vi "guangzi - 可控采集.vi"() -> ()   [LabVIEW 2016]
uses:
  <vilib>/Utility/file.llb/Write To Spreadsheet File (DBL).vi
panel:
  in  "采集记录开关":bool
  out "切片图":u32[](graph)
  in  "切片值":i32
  in  "选项卡控件":T1(tab)
  in  "对数":bool
  out "MCS8Dat Error":i32
  out "CHN Status":T2 {"Dummy" format="%.2f"; "Starts" format="%.2f"; "Sweeps" format="%.2f"; "Roirate" format="%.2f"; "RoiSum" format="%.2f"; "TotalSum" format="%.2f"; "Fifo full" format="%.2f"; "Runtime" format="%.2f"}
  out "Data":u32[](graph)
  out "Settings":T3 {"dummy3" format="%.2f"; "dummy2" format="%.2f"; "bitshift" format="%.0x"; "Active" format="%.0x"; "Offset" format="%.0x"; "Param" format="%.0x"; "dummy1" format="%.2f"; "Roipreset" format="%.2f"; "cftfak" format="%.0x"}
  out "通道数":i32
  out "Data 9":dbl[](graph)
  out "Data 2":u32[](graph)
  out "MCS8Dat Error 2":i32
  out "Settings 2":T3 {"dummy3" format="%.2f"; "dummy2" format="%.2f"; "bitshift" format="%.0x"; "Active" format="%.0x"; "Offset" format="%.0x"; "Param" format="%.0x"; "dummy1" format="%.2f"; "Roipreset" format="%.2f"; "cftfak" format="%.0x"}
  out "CHN Status 2":T2 {"Dummy" format="%.2f"; "Starts" format="%.2f"; "Sweeps" format="%.2f"; "Roirate" format="%.2f"; "RoiSum" format="%.2f"; "TotalSum" format="%.2f"; "Fifo full" format="%.2f"; "Runtime" format="%.2f"}
  out "通道数 2":i32
  in  "对数 2":bool
  out "Data10":dbl[](graph)
  out "Data 3":u32[](graph)
  out "MCS8Dat Error 3":i32
  out "Settings 3":T3 {"dummy3" format="%.2f"; "dummy2" format="%.2f"; "bitshift" format="%.0x"; "Active" format="%.0x"; "Offset" format="%.0x"; "Param" format="%.0x"; "dummy1" format="%.2f"; "Roipreset" format="%.2f"; "cftfak" format="%.0x"}
  out "CHN Status 3":T2 {"Dummy" format="%.2f"; "Starts" format="%.2f"; "Sweeps" format="%.2f"; "Roirate" format="%.2f"; "RoiSum" format="%.2f"; "TotalSum" format="%.2f"; "Fifo full" format="%.2f"; "Runtime" format="%.2f"}
  out "通道数 3":i32
  in  "对数 3":bool
  out "Data10 2":dbl[](graph)
  out "Data 4":u32[](graph)
  out "MCS8Dat Error 4":i32
  out "Settings 4":T3 {"dummy3" format="%.2f"; "dummy2" format="%.2f"; "bitshift" format="%.0x"; "Active" format="%.0x"; "Offset" format="%.0x"; "Param" format="%.0x"; "dummy1" format="%.2f"; "Roipreset" format="%.2f"; "cftfak" format="%.0x"}
  out "CHN Status 4":T2 {"Dummy" format="%.2f"; "Starts" format="%.2f"; "Sweeps" format="%.2f"; "Roirate" format="%.2f"; "RoiSum" format="%.2f"; "TotalSum" format="%.2f"; "Fifo full" format="%.2f"; "Runtime" format="%.2f"}
  out "通道数 4":i32
  in  "对数 4":bool
  out "Data10 3":dbl[](graph)
  out "Data 5":u32[](graph)
  out "MCS8Dat Error 5":i32
  out "Settings 5":T3 {"dummy3" format="%.2f"; "dummy2" format="%.2f"; "bitshift" format="%.0x"; "Active" format="%.0x"; "Offset" format="%.0x"; "Param" format="%.0x"; "dummy1" format="%.2f"; "Roipreset" format="%.2f"; "cftfak" format="%.0x"}
  out "CHN Status 5":T2 {"Dummy" format="%.2f"; "Starts" format="%.2f"; "Sweeps" format="%.2f"; "Roirate" format="%.2f"; "RoiSum" format="%.2f"; "TotalSum" format="%.2f"; "Fifo full" format="%.2f"; "Runtime" format="%.2f"}
  out "通道数 5":i32
  in  "对数 5":bool
  out "Data10 4":dbl[](graph)
  out "Data 6":u32[](graph)
  out "MCS8Dat Error 6":i32
  out "Settings 6":T3 {"dummy3" format="%.2f"; "dummy2" format="%.2f"; "bitshift" format="%.0x"; "Active" format="%.0x"; "Offset" format="%.0x"; "Param" format="%.0x"; "dummy1" format="%.2f"; "Roipreset" format="%.2f"; "cftfak" format="%.0x"}
  out "CHN Status 6":T2 {"Dummy" format="%.2f"; "Starts" format="%.2f"; "Sweeps" format="%.2f"; "Roirate" format="%.2f"; "RoiSum" format="%.2f"; "TotalSum" format="%.2f"; "Fifo full" format="%.2f"; "Runtime" format="%.2f"}
  out "通道数 6":i32
  in  "对数 6":bool
  out "Data10 5":dbl[](graph)
  out "Data 7":u32[](graph)
  out "MCS8Dat Error 7":i32
  out "Settings 7":T3 {"dummy3" format="%.2f"; "dummy2" format="%.2f"; "bitshift" format="%.0x"; "Active" format="%.0x"; "Offset" format="%.0x"; "Param" format="%.0x"; "dummy1" format="%.2f"; "Roipreset" format="%.2f"; "cftfak" format="%.0x"}
  out "CHN Status 7":T2 {"Dummy" format="%.2f"; "Starts" format="%.2f"; "Sweeps" format="%.2f"; "Roirate" format="%.2f"; "RoiSum" format="%.2f"; "TotalSum" format="%.2f"; "Fifo full" format="%.2f"; "Runtime" format="%.2f"}
  out "通道数 7":i32
  in  "对数 7":bool
  out "Data10 6":dbl[](graph)
  out "Data 8":u32[](graph)
  out "MCS8Dat Error 8":i32
  out "Settings 8":T3 {"dummy3" format="%.2f"; "dummy2" format="%.2f"; "bitshift" format="%.0x"; "Active" format="%.0x"; "Offset" format="%.0x"; "Param" format="%.0x"; "dummy1" format="%.2f"; "Roipreset" format="%.2f"; "cftfak" format="%.0x"}
  out "CHN Status 8":T2 {"Dummy" format="%.2f"; "Starts" format="%.2f"; "Sweeps" format="%.2f"; "Roirate" format="%.2f"; "RoiSum" format="%.2f"; "TotalSum" format="%.2f"; "Fifo full" format="%.2f"; "Runtime" format="%.2f"}
  out "通道数 8":i32
  in  "对数 8":bool
  out "Data10 7":dbl[](graph)
  in  "子开关":bool
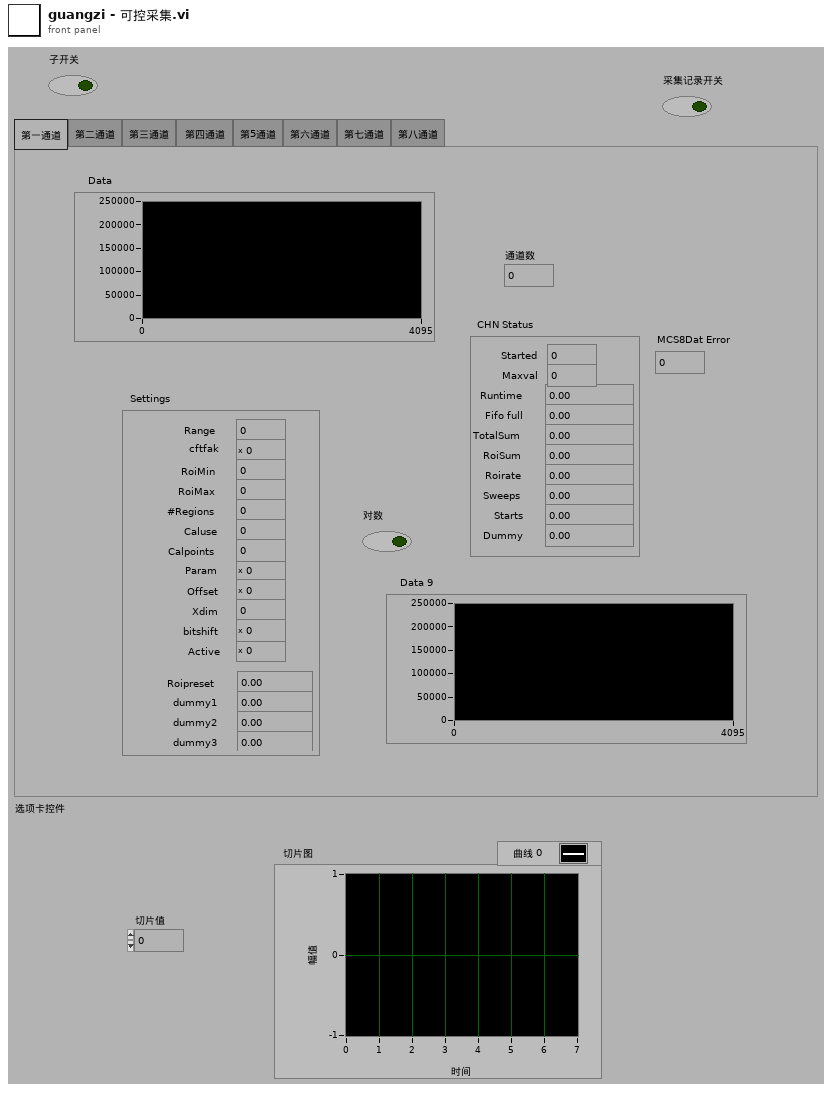
[diagram p1: front panel]
types:
  T1 = enum32{"第一通道", "第二通道", "第三通道", "第四通道 ", "第5通道", "第六通道", "第七通道", "第八通道"}
  T2 = cluster{"Started":i32, "Maxval":u32, "Runtime":dbl, "Fifo full":dbl, "TotalSum":dbl, "RoiSum":dbl, "Roirate":dbl, "Sweeps":dbl, "Starts":dbl, "Dummy":dbl}
  T3 = cluster{"Range":i32, "cftfak":i32, "RoiMin":i32, "RoiMax":i32, "#Regions":i32, "Caluse":i32, "Calpoints":i32, "Param":i32, "Offset":i32, "Xdim":i32, "bitshift":i32, "Active":i32, "Roipreset":dbl, "dummy1":dbl, "dummy2":dbl, "dummy3":dbl}
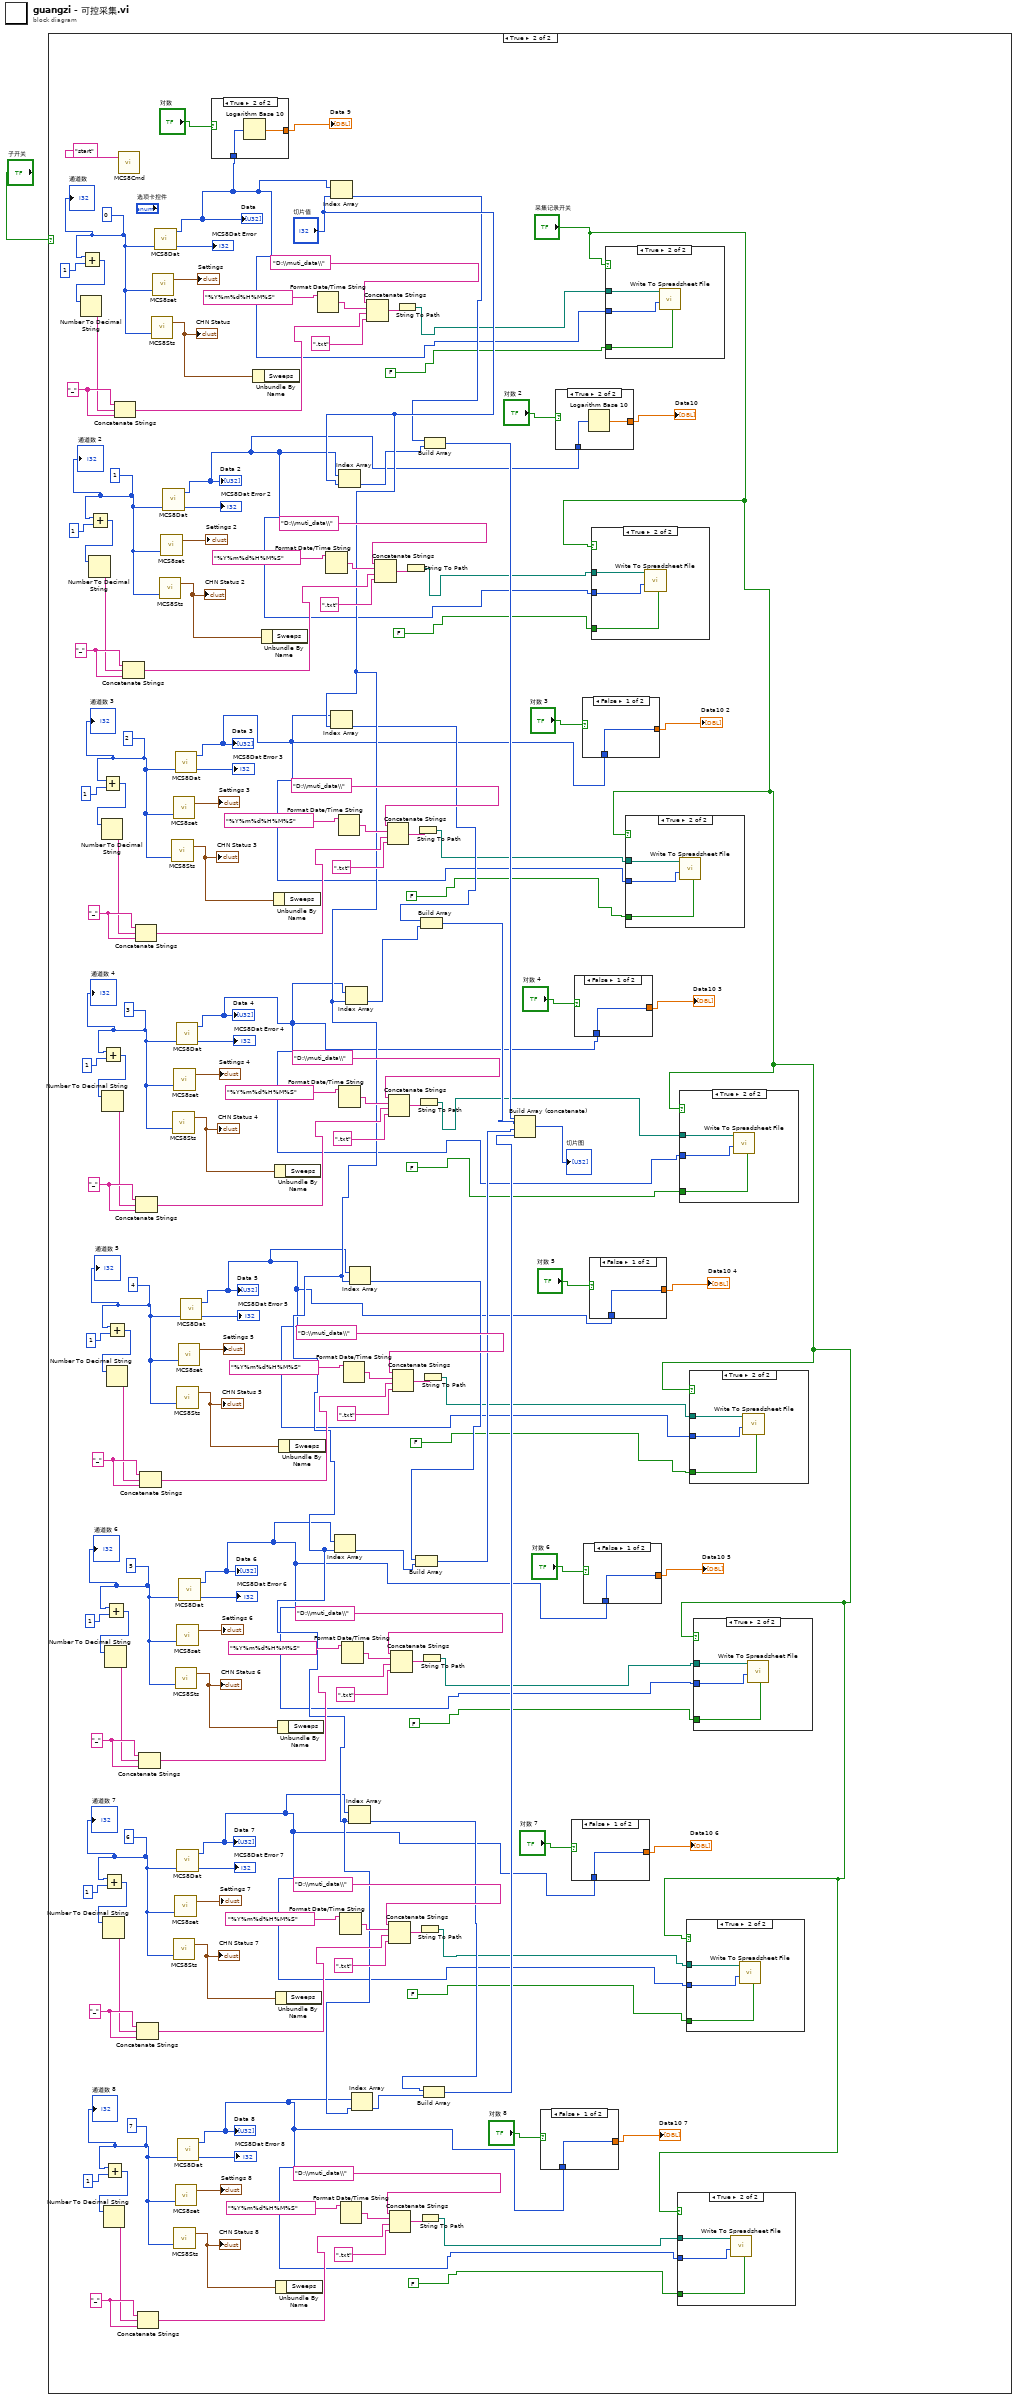
[diagram p0: block diagram]
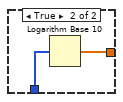
[diagram p11: hidden frame]
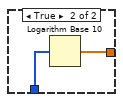
[diagram p12: hidden frame]
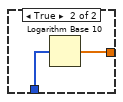
[diagram p13: hidden frame]
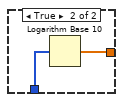
[diagram p14: hidden frame]
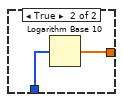
[diagram p15: hidden frame]
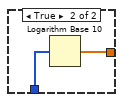
[diagram p16: hidden frame]
diagram:
  n1 = case shown="True" "子开关" {
    frame False {
    }
    frame True {
      w57 = 7
      w65 = "_"
      w71 = 6
      w79 = "_"
      w85 = 5
      w93 = "_"
      w99 = 4
      w107 = "_"
      w113 = 3
      w121 = "_"
      w127 = 2
      w135 = "_"
      w141 = 1
      w149 = "_"
      w155 = 0
      w163 = "_"
      n2 = Add(x=w155, y=1) -> (x+y=w158:i32)
      n3 = Number To Decimal String(number=w158) -> (decimal integer string=w162:string)  [unwired: 1 in]
      n4 = Add(x=w141, y=1) -> (x+y=w144:i32)
      n5 = Number To Decimal String(number=w144) -> (decimal integer string=w148:string)  [unwired: 1 in]
      n6 = Add(x=w127, y=1) -> (x+y=w130:i32)
      n7 = Number To Decimal String(number=w130) -> (decimal integer string=w134:string)  [unwired: 1 in]
      n8 = Add(x=w113, y=1) -> (x+y=w116:i32)
      n9 = Number To Decimal String(number=w116) -> (decimal integer string=w120:string)  [unwired: 1 in]
      n10 = Add(x=w71, y=1) -> (x+y=w74:i32)
      n11 = Number To Decimal String(number=w74) -> (decimal integer string=w78:string)  [unwired: 1 in]
      n12 = Add(x=w57, y=1) -> (x+y=w60:i32)
      n13 = Number To Decimal String(number=w60) -> (decimal integer string=w64:string)  [unwired: 1 in]
      n14 = Add(x=w85, y=1) -> (x+y=w88:i32)
      n15 = Number To Decimal String(number=w88) -> (decimal integer string=w92:string)  [unwired: 1 in]
      n16 = Add(x=w99, y=1) -> (x+y=w102:i32)
      n17 = Number To Decimal String(number=w102) -> (decimal integer string=w106:string)  [unwired: 1 in]
      n18 = Concatenate Strings(w163, w162, w163) -> (w161:string)
      n19 = call "MCS8Cmd.vi"("Command"="start") -> ()  [unwired: 2 in, 1 out]
      n20 = Concatenate Strings(w149, w148, w149) -> (w147:string)
      n21 = Concatenate Strings(w135, w134, w135) -> (w133:string)
      n22 = Concatenate Strings(w121, w120, w121) -> (w119:string)
      n23 = Concatenate Strings(w79, w78, w79) -> (w77:string)
      n24 = Concatenate Strings(w65, w64, w65) -> (w63:string)
      n25 = Concatenate Strings(w93, w92, w93) -> (w91:string)
      n26 = Concatenate Strings(w107, w106, w107) -> (w105:string)
      n27 = call "MCS8Sts.vi"("CHN #"=w155) -> ("CHN Status"=w168:T2)  [unwired: 1 in, 1 out]
      "CHN Status" <- w168
      n28 = call "MCS8set.vi"("Spect #"=w155) -> ("Settings"=→"Settings":T3)  [unwired: 1 in, 1 out]
      n29 = call "MCS8Dat.vi"("Spectrum #"=w155) -> ("MCS8Dat Error"=→"MCS8Dat Error":i32, "Data"=w25:u32[])  [unwired: 2 in, 1 out]
      "Data" <- w25
      n30 = call "MCS8Sts.vi"("CHN #"=w141) -> ("CHN Status"=w154:T2)  [unwired: 1 in, 1 out]
      "CHN Status 2" <- w154
      n31 = call "MCS8set.vi"("Spect #"=w141) -> ("Settings"=→"Settings 2":T3)  [unwired: 1 in, 1 out]
      n32 = call "MCS8Dat.vi"("Spectrum #"=w141) -> ("MCS8Dat Error"=→"MCS8Dat Error 2":i32, "Data"=w22:u32[])  [unwired: 2 in, 1 out]
      "Data 2" <- w22
      n33 = call "MCS8Sts.vi"("CHN #"=w127) -> ("CHN Status"=w140:T2)  [unwired: 1 in, 1 out]
      "CHN Status 3" <- w140
      n34 = call "MCS8Sts.vi"("CHN #"=w113) -> ("CHN Status"=w126:T2)  [unwired: 1 in, 1 out]
      "CHN Status 4" <- w126
      n35 = call "MCS8set.vi"("Spect #"=w127) -> ("Settings"=→"Settings 3":T3)  [unwired: 1 in, 1 out]
      n36 = call "MCS8Sts.vi"("CHN #"=w71) -> ("CHN Status"=w84:T2)  [unwired: 1 in, 1 out]
      "CHN Status 7" <- w84
      n37 = call "MCS8set.vi"("Spect #"=w113) -> ("Settings"=→"Settings 4":T3)  [unwired: 1 in, 1 out]
      n38 = call "MCS8Sts.vi"("CHN #"=w57) -> ("CHN Status"=w70:T2)  [unwired: 1 in, 1 out]
      "CHN Status 8" <- w70
      n39 = call "MCS8set.vi"("Spect #"=w71) -> ("Settings"=→"Settings 7":T3)  [unwired: 1 in, 1 out]
      n40 = call "MCS8Dat.vi"("Spectrum #"=w127) -> ("MCS8Dat Error"=→"MCS8Dat Error 3":i32, "Data"=w19:u32[])  [unwired: 2 in, 1 out]
      "Data 3" <- w19
      n41 = call "MCS8Sts.vi"("CHN #"=w85) -> ("CHN Status"=w98:T2)  [unwired: 1 in, 1 out]
      "CHN Status 6" <- w98
      n42 = call "MCS8set.vi"("Spect #"=w57) -> ("Settings"=→"Settings 8":T3)  [unwired: 1 in, 1 out]
      n43 = call "MCS8Dat.vi"("Spectrum #"=w113) -> ("MCS8Dat Error"=→"MCS8Dat Error 4":i32, "Data"=w15:u32[])  [unwired: 2 in, 1 out]
      "Data 4" <- w15
      n44 = call "MCS8Sts.vi"("CHN #"=w99) -> ("CHN Status"=w112:T2)  [unwired: 1 in, 1 out]
      "CHN Status 5" <- w112
      n45 = call "MCS8set.vi"("Spect #"=w85) -> ("Settings"=→"Settings 6":T3)  [unwired: 1 in, 1 out]
      n46 = call "MCS8Dat.vi"("Spectrum #"=w71) -> ("MCS8Dat Error"=→"MCS8Dat Error 7":i32, "Data"=w7:u32[])  [unwired: 2 in, 1 out]
      "Data 7" <- w7
      n47 = call "MCS8Dat.vi"("Spectrum #"=w57) -> ("MCS8Dat Error"=→"MCS8Dat Error 8":i32, "Data"=w3:u32[])  [unwired: 2 in, 1 out]
      "Data 8" <- w3
      n48 = call "MCS8set.vi"("Spect #"=w99) -> ("Settings"=→"Settings 5":T3)  [unwired: 1 in, 1 out]
      n49 = call "MCS8Dat.vi"("Spectrum #"=w85) -> ("MCS8Dat Error"=→"MCS8Dat Error 6":i32, "Data"=w10:u32[])  [unwired: 2 in, 1 out]
      "Data 6" <- w10
      n50 = call "MCS8Dat.vi"("Spectrum #"=w99) -> ("MCS8Dat Error"=→"MCS8Dat Error 5":i32, "Data"=w13:u32[])  [unwired: 2 in, 1 out]
      "Data 5" <- w13
      n51 = case shown="True" "对数" {
        tunnel: w25 -> [w215 w217]
        tunnel: [w215 w216] -> w41
        frame False {
        }
        frame True {
          n52 = Logarithm Base 10(1:w217) -> (0:w216:dbl[])
        }
      }
      "Data 9" <- w41
      n53 = Unbundle By Name(w168) -> ()  [unwired: 1 out]
      n54 = Unbundle By Name(w154) -> ()  [unwired: 1 out]
      n55 = Unbundle By Name(w140) -> ()  [unwired: 1 out]
      n56 = Unbundle By Name(w126) -> ()  [unwired: 1 out]
      n57 = Unbundle By Name(w84) -> ()  [unwired: 1 out]
      n58 = Unbundle By Name(w70) -> ()  [unwired: 1 out]
      n59 = Unbundle By Name(w98) -> ()  [unwired: 1 out]
      n60 = Unbundle By Name(w112) -> ()  [unwired: 1 out]
      n61 = Format Date/Time String(time format string (%c)="%Y%m%d%H%M%S") -> (date/time string=w159:string)  [unwired: 2 in]
      n62 = Format Date/Time String(time format string (%c)="%Y%m%d%H%M%S") -> (date/time string=w145:string)  [unwired: 2 in]
      n63 = Index Array(array=w25, index="切片值") -> (element=w49:u32)
      n64 = Index Array(array=w19, index="切片值") -> (element=w51:u32)
      n65 = Index Array(array=w10, index="切片值") -> (element=w53:u32)
      n66 = Format Date/Time String(time format string (%c)="%Y%m%d%H%M%S") -> (date/time string=w131:string)  [unwired: 2 in]
      n67 = Index Array(array=w22, index="切片值") -> (element=w48:u32)
      n68 = Format Date/Time String(time format string (%c)="%Y%m%d%H%M%S") -> (date/time string=w117:string)  [unwired: 2 in]
      n69 = Format Date/Time String(time format string (%c)="%Y%m%d%H%M%S") -> (date/time string=w75:string)  [unwired: 2 in]
      n70 = Format Date/Time String(time format string (%c)="%Y%m%d%H%M%S") -> (date/time string=w61:string)  [unwired: 2 in]
      n71 = Format Date/Time String(time format string (%c)="%Y%m%d%H%M%S") -> (date/time string=w89:string)  [unwired: 2 in]
      n72 = Format Date/Time String(time format string (%c)="%Y%m%d%H%M%S") -> (date/time string=w103:string)  [unwired: 2 in]
      n73 = Index Array(array=w15, index="切片值") -> (element=w50:u32)
      n74 = Index Array(array=w7, index="切片值") -> (element=w54:u32)
      n75 = Index Array(array=w13, index="切片值") -> (element=w52:u32)
      n76 = Index Array(array=w3, index="切片值") -> (element=w55:u32)
      n77 = Concatenate Strings("D:\\muti_data\\", w159, w161, ".txt") -> (w165:string)
      n78 = Concatenate Strings("D:\\muti_data\\", w145, w147, ".txt") -> (w151:string)
      n79 = Concatenate Strings("D:\\muti_data\\", w131, w133, ".txt") -> (w137:string)
      n80 = Concatenate Strings("D:\\muti_data\\", w117, w119, ".txt") -> (w123:string)
      n81 = Concatenate Strings("D:\\muti_data\\", w75, w77, ".txt") -> (w81:string)
      n82 = Concatenate Strings("D:\\muti_data\\", w61, w63, ".txt") -> (w67:string)
      n83 = Concatenate Strings("D:\\muti_data\\", w89, w91, ".txt") -> (w95:string)
      n84 = Concatenate Strings("D:\\muti_data\\", w103, w105, ".txt") -> (w109:string)
      n85 = String To Path(string=w165) -> (path=w26:path)
      n86 = String To Path(string=w151) -> (path=w23:path)
      n87 = Build Array(w52, w53) -> (w45:u32[])
      n88 = String To Path(string=w137) -> (path=w20:path)
      n89 = String To Path(string=w123) -> (path=w17:path)
      n90 = String To Path(string=w81) -> (path=w8:path)
      n91 = String To Path(string=w67) -> (path=w4:path)
      n92 = Build Array(w51, w50) -> (w46:u32[])
      n93 = String To Path(string=w95) -> (path=w11:path)
      n94 = String To Path(string=w109) -> (path=w14:path)
      n95 = Build Array(w54, w55) -> (w44:u32[])
      n96 = Build Array(w49, w48) -> (w47:u32[])
      n97 = Build Array (concatenate)(w47, w46, w45, w44) -> (→"切片图":u32[])
      n98 = case shown="False" "对数 8" {
        tunnel: w3 -> [w194 w196]
        tunnel: [w194 w195] -> w27
        frame False {
        }
        frame True {
          n99 = Logarithm Base 10(1:w196) -> (0:w195:dbl[])
        }
      }
      "Data10 7" <- w27
      n100 = case shown="True" "对数 2" {
        tunnel: w22 -> [w212 w214]
        tunnel: [w212 w213] -> w39
        frame False {
        }
        frame True {
          n101 = Logarithm Base 10(1:w214) -> (0:w213:dbl[])
        }
      }
      "Data10" <- w39
      n102 = case shown="False" "对数 7" {
        tunnel: w7 -> [w197 w199]
        tunnel: [w197 w198] -> w29
        frame False {
        }
        frame True {
          n103 = Logarithm Base 10(1:w199) -> (0:w198:dbl[])
        }
      }
      "Data10 6" <- w29
      n104 = case shown="False" "对数 4" {
        tunnel: w15 -> [w206 w208]
        tunnel: [w206 w207] -> w35
        frame False {
        }
        frame True {
          n105 = Logarithm Base 10(1:w208) -> (0:w207:dbl[])
        }
      }
      "Data10 3" <- w35
      n106 = case shown="False" "对数 3" {
        tunnel: w19 -> [w209 w211]
        tunnel: [w209 w210] -> w37
        frame False {
        }
        frame True {
          n107 = Logarithm Base 10(1:w211) -> (0:w210:dbl[])
        }
      }
      "Data10 2" <- w37
      n108 = case shown="False" "对数 6" {
        tunnel: w10 -> [w200 w202]
        tunnel: [w200 w201] -> w31
        frame False {
        }
        frame True {
          n109 = Logarithm Base 10(1:w202) -> (0:w201:dbl[])
        }
      }
      "Data10 5" <- w31
      n110 = case shown="False" "对数 5" {
        tunnel: w13 -> [w203 w205]
        tunnel: [w203 w204] -> w33
        frame False {
        }
        frame True {
          n111 = Logarithm Base 10(1:w205) -> (0:w204:dbl[])
        }
      }
      "Data10 4" <- w33
      n112 = case shown="True" "采集记录开关" {
        tunnel: w23 -> [_ w190]
        tunnel: w22 -> [_ w189]
        tunnel: FALSE -> [_ w188]
        frame False {
        }
        frame True {
          n113 = call-poly <vilib>:"Write To Spreadsheet File.vi"("transpose? (no:F)"=w188, "1D data"=w189, "file path (dialog if empty)"=w190) -> ()  [unwired: 5 in, 1 out]
        }
      }
      n114 = case shown="True" "采集记录开关" {
        tunnel: w26 -> [_ w193]
        tunnel: w25 -> [_ w192]
        tunnel: FALSE -> [_ w191]
        frame False {
        }
        frame True {
          n115 = call-poly <vilib>:"Write To Spreadsheet File.vi"("transpose? (no:F)"=w191, "1D data"=w192, "file path (dialog if empty)"=w193) -> ()  [unwired: 5 in, 1 out]
        }
      }
      n116 = case shown="True" "采集记录开关" {
        tunnel: w20 -> [_ w187]
        tunnel: w19 -> [_ w186]
        tunnel: FALSE -> [_ w185]
        frame False {
        }
        frame True {
          n117 = call-poly <vilib>:"Write To Spreadsheet File.vi"("transpose? (no:F)"=w185, "1D data"=w186, "file path (dialog if empty)"=w187) -> ()  [unwired: 5 in, 1 out]
        }
      }
      n118 = case shown="True" "采集记录开关" {
        tunnel: w4 -> [_ w172]
        tunnel: w3 -> [_ w171]
        tunnel: FALSE -> [_ w170]
        frame False {
        }
        frame True {
          n119 = call-poly <vilib>:"Write To Spreadsheet File.vi"("transpose? (no:F)"=w170, "1D data"=w171, "file path (dialog if empty)"=w172) -> ()  [unwired: 5 in, 1 out]
        }
      }
      n120 = case shown="True" "采集记录开关" {
        tunnel: w17 -> [_ w184]
        tunnel: w15 -> [_ w183]
        tunnel: FALSE -> [_ w182]
        frame False {
        }
        frame True {
          n121 = call-poly <vilib>:"Write To Spreadsheet File.vi"("transpose? (no:F)"=w182, "1D data"=w183, "file path (dialog if empty)"=w184) -> ()  [unwired: 5 in, 1 out]
        }
      }
      n122 = case shown="True" "采集记录开关" {
        tunnel: w8 -> [_ w175]
        tunnel: w7 -> [_ w174]
        tunnel: FALSE -> [_ w173]
        frame False {
        }
        frame True {
          n123 = call-poly <vilib>:"Write To Spreadsheet File.vi"("transpose? (no:F)"=w173, "1D data"=w174, "file path (dialog if empty)"=w175) -> ()  [unwired: 5 in, 1 out]
        }
      }
      n124 = case shown="True" "采集记录开关" {
        tunnel: w14 -> [_ w181]
        tunnel: w13 -> [_ w180]
        tunnel: FALSE -> [_ w179]
        frame False {
        }
        frame True {
          n125 = call-poly <vilib>:"Write To Spreadsheet File.vi"("transpose? (no:F)"=w179, "1D data"=w180, "file path (dialog if empty)"=w181) -> ()  [unwired: 5 in, 1 out]
        }
      }
      n126 = case shown="True" "采集记录开关" {
        tunnel: w11 -> [_ w178]
        tunnel: w10 -> [_ w177]
        tunnel: FALSE -> [_ w176]
        frame False {
        }
        frame True {
          n127 = call-poly <vilib>:"Write To Spreadsheet File.vi"("transpose? (no:F)"=w176, "1D data"=w177, "file path (dialog if empty)"=w178) -> ()  [unwired: 5 in, 1 out]
        }
      }
      "通道数" <- w155
      "通道数 2" <- w141
      "通道数 3" <- w127
      "通道数 4" <- w113
      "通道数 5" <- w99
      "通道数 6" <- w85
      "通道数 7" <- w71
      "通道数 8" <- w57
    }
  }
